vi "tempSensorProcs.vi"(0 "frame":u8[](array[numeric])) -> ()   [LabVIEW 2021]
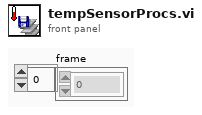
[diagram p1: front panel]
types:
  T1 = cluster{"ValvePos1":sgl, "ValvePos2":sgl, "PressureArray":sgl[], "TempArray2":sgl[], "TempArray1":sgl[], "Valve 1 Time Stamp":timestamp, "Temp 2 Array Time Stamp":timestamp[], "Temp 1 Array Time Stamp":timestamp[], "Valve 2 Time Stamp":timestamp, "Press Array Time Stamp":timestamp[]}
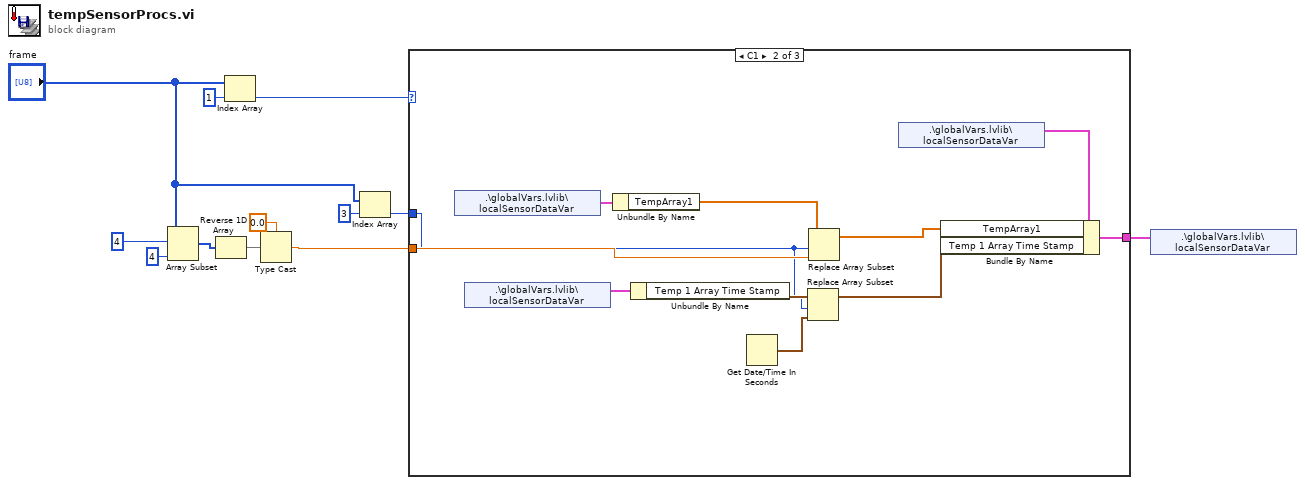
[diagram p0: block diagram]
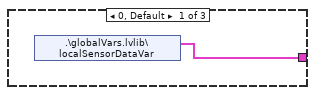
[diagram p2: hidden frame]
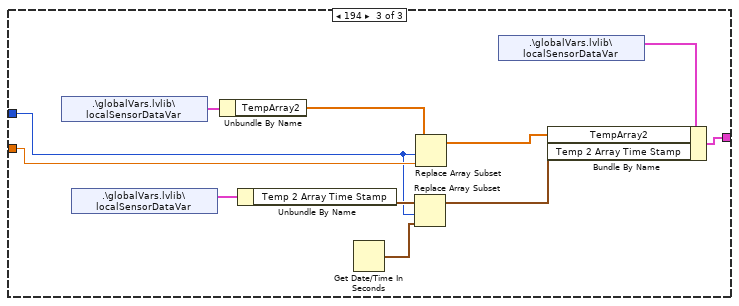
[diagram p3: hidden frame]
diagram:
  n1 = Array Subset(array="frame", index=4, length=4) -> (w10:u8[])
  n2 = Reverse 1D Array(array=w10) -> (reversed array=w11:u8[])
  n3 = Index Array(array="frame", index=1) -> (element=w5:u8)
  n4 = Type Cast(type=sgl 0.0, x=w11) -> (*(type *) &x=w4:sgl)
  n5 = Index Array(array="frame", index=3) -> (element=w1:u8)
  n6 = case shown="C1" w5 {
    tunnel: [w13 w21 w28] -> w6
    tunnel: w4 -> [_ w16 w29]
    tunnel: w1 -> [_ w14 w25]
    frame 0, Default {
      n7 = shared-variable ".\\globalVars.lvlib\\localSensorDataVar"() -> (w13:T1)  [unwired: 1 in, 1 out]
    }
    frame 193 {
      n8 = shared-variable ".\\globalVars.lvlib\\localSensorDataVar"() -> (w24:T1)  [unwired: 1 in, 1 out]
      n9 = shared-variable ".\\globalVars.lvlib\\localSensorDataVar"() -> (w20:T1)  [unwired: 1 in, 1 out]
      n10 = Unbundle By Name(w24) -> ("TempArray1"=w23:sgl[])
      n11 = Unbundle By Name(w20) -> ("Temp 1 Array Time Stamp"=w18:timestamp[])
      n12 = Get Date/Time In Seconds() -> (seconds since 1Jan1904=w19:timestamp)
      n13 = Replace Array Subset(array=w18, new element=w19, index=w14) -> (w17:timestamp[])
      n14 = Replace Array Subset(array=w23, new element=w16, index=w14) -> (w22:sgl[])
      n15 = shared-variable ".\\globalVars.lvlib\\localSensorDataVar"() -> (w15:T1)  [unwired: 1 in, 1 out]
      n16 = Bundle By Name(cluster=w15, "TempArray1"=w22, "Temp 1 Array Time Stamp"=w17) -> (w21:T1)
    }
    frame 194 {
      n17 = shared-variable ".\\globalVars.lvlib\\localSensorDataVar"() -> (w35:T1)  [unwired: 1 in, 1 out]
      n18 = shared-variable ".\\globalVars.lvlib\\localSensorDataVar"() -> (w32:T1)  [unwired: 1 in, 1 out]
      n19 = Unbundle By Name(w35) -> ("TempArray2"=w34:sgl[])
      n20 = Unbundle By Name(w32) -> ("Temp 2 Array Time Stamp"=w31:timestamp[])
      n21 = Get Date/Time In Seconds() -> (seconds since 1Jan1904=w26:timestamp)
      n22 = Replace Array Subset(array=w31, new element=w26, index=w25) -> (w30:timestamp[])
      n23 = Replace Array Subset(array=w34, new element=w29, index=w25) -> (w33:sgl[])
      n24 = shared-variable ".\\globalVars.lvlib\\localSensorDataVar"() -> (w27:T1)  [unwired: 1 in, 1 out]
      n25 = Bundle By Name(cluster=w27, "TempArray2"=w33, "Temp 2 Array Time Stamp"=w30) -> (w28:T1)
    }
  }
  n26 = shared-variable ".\\globalVars.lvlib\\localSensorDataVar"(w6) -> ()  [unwired: 1 in, 1 out]
